vi "InterpolateCalibrationValue.vi"(1 "Input":dbl, 2 "Calibration Data":dbl[][](array[numeric])) -> (0 "Interpolated Output":dbl)   [LabVIEW 2019]
doc: "Estimates a value using linear interpolation. This VI is configured to work with the FRC 4265 standard for sensor calibration files."
uses:
  <vilib>/gmath/NI_Gmath.lvlib
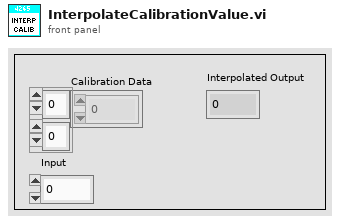
[diagram p1: front panel]
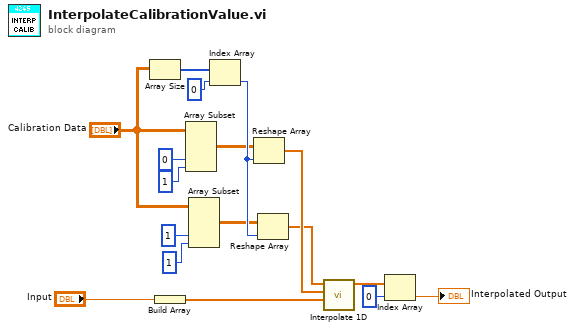
[diagram p0: block diagram]
diagram:
  n1 = Array Size(array="Calibration Data") -> (size(s)=w14:i32[])
  n2 = Build Array("Input") -> (w5:dbl[])
  n3 = Array Subset(array="Calibration Data", index (col)=0 ("index"), length (col)=1 ("length")) -> (w11:dbl[][])  [unwired: 2 in]
  n4 = Array Subset(array="Calibration Data", index (col)=1 ("index"), length (col)=1 ("length")) -> (w15:dbl[][])  [unwired: 2 in]
  n5 = Index Array(array=w14, index=0) -> (element=w16:i32)
  n6 = Reshape Array(w11, w16) -> (w2:dbl[])
  n7 = Reshape Array(w15, w16) -> (w1:dbl[])
  n8 = call <vilib>:"Interpolate 1D.vi"("xi"=w5, "X"=w2, "Y"=w1) -> ("yi"=w4:dbl[])  [unwired: 6 in, 2 out]
  n9 = Index Array(array=w4, index=0) -> (element=→"Interpolated Output":dbl)
